vi "http check to close connection.vi"(11 "application request":T1) -> (1 "leave connection open?":bool, 2 "stop process?":bool, 3 "application request out":T1)   [LabVIEW 2013]
uses:
  http response.ctl
  http response packet type.ctl
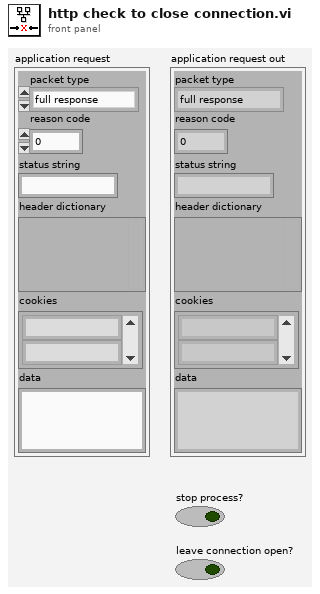
[diagram p1: front panel]
types:
  T1 = typedef "http response.ctl" = cluster{"packet type":T2, "reason code":u16, "status string":string, "header dictionary":variant, "cookies":string[], "data":string}
  T2 = typedef "http response packet type.ctl" = enum16{"full response", "header only", "data only", "last data"}
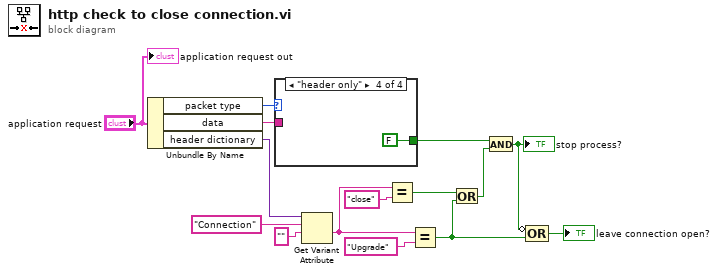
[diagram p0: block diagram]
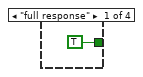
[diagram p2: hidden frame]
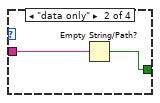
[diagram p3: hidden frame]
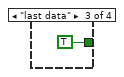
[diagram p4: hidden frame]
diagram:
  n1 = Unbundle By Name("application request") -> ("packet type"=w9:T2, "data"=w7:string, "header dictionary"=w13:variant)
  n2 = case shown="\"header only\"" w9 {
    tunnel: [TRUE w17 TRUE FALSE] -> w8
    tunnel: w7 -> [_ w18 _ _]
    frame "full response" {
    }
    frame "data only" {
      n3 = Empty String/Path?(string/path=w18) -> (empty?=w17:bool)
    }
    frame "last data" {
    }
    frame "header only" {
    }
  }
  n4 = Get Variant Attribute(Variant=w13, name="Connection", default value (empty Variant)="" ("name")) -> (value=w5:string)  [unwired: 1 in, 3 out]
  n5 = Equal?(x=w5, y="close" ("name")) -> (x = y?=w15:bool)
  n6 = Equal?(x=w5, y="Upgrade" ("name")) -> (x = y?=w1:bool)
  n7 = Or(x=w15, y=w1) -> (x .or. y?=w2:bool)
  n8 = And(x=w8, y=w2) -> (x .and. y?=w4:bool)
  "stop process?" <- w4
  n9 = Compound Arithmetic op=OR(invert w4, w1) -> (→"leave connection open?":bool)
  "application request out" <- "application request"
